vi "Set Scaling Factor.vi"(8 "error in (no error)":errorcluster, 10 "Value":sgl, 11 "WeChat QR Code Detector in":refnum<class "WeChat QR Code Detector.lvclass">) -> (0 "error out":errorcluster, 3 "WeChat QR Code Detector":refnum<class "WeChat QR Code Detector.lvclass">)   [LabVIEW 2020, in "feature_detection.lvlib" / "WeChat QR Code Detector.lvclass"]
doc: "Set the scaling factor to apply to the image before processing. Use a value between 0 and 1.\n\nA value of -1 means to automatically set the scaling factor to give an image area of 160000 pixels."
uses:
  WeChat QR Code Detector.lvclass
  WeChat QR Code Detector.lvclass/WeChat QR Code Detector.ctl
  <vilib>/Utility/error.llb/Error Cluster From Error Code.vi
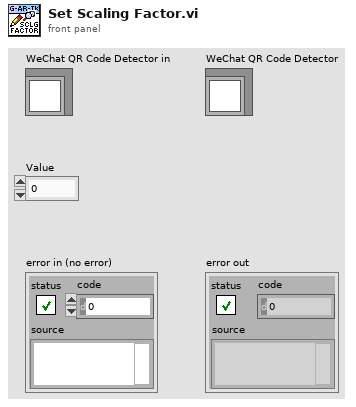
[diagram p1: front panel]
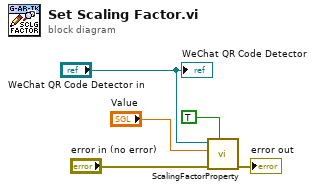
[diagram p0: block diagram]
diagram:
  n1 = call "ScalingFactorProperty.vi"("Write?"=TRUE, "error in (no error)"="error in (no error)", "Value in"="Value", "QR Code Detector in"="WeChat QR Code Detector in") -> ("error out"=→"error out":errorcluster)  [unwired: 6 in, 1 out]
  "WeChat QR Code Detector" <- "WeChat QR Code Detector in"
